vi "Load 1PLOT.vi"(8 "error in (no error)":errorcluster, 11 "Config Ops":T6={"file extension"="", "start path"=path ""}) -> (0 "error out":errorcluster, 2 "Valid load?":bool, 3 "Plot Config":T1={"plots"=[], "X-axis"={"Name Label.Text"="", "Style"=0, "Tick Colors:Minor Tick Color"=0, "Tick Colors:Tick Color"=0, "Marker Colors:Text Color"=0, "Grid Colors:Major Color"=0, "Grid Colors:Minor Color"=0, "Mapping Mode"=0, "Flipped"=FALSE, "Name Label.Visible"=FALSE, "Name Label.Text Colors:Text Color"=0, "Scale Fit"=0, "Range:Maximum"=0.0, "Range:Minimum"=0.0, "Offset and Multiplier:Multiplier"=0.0, "Offset and Multiplier:Offset"=0.0, "Name Label.Font:Size"=0, "Marker.Font:Size"=0, "Uniform Marker Spacing?"=TRUE, "Format String"=""}, "Y-axes"=[], "General"={"Title"="", "Time to Plot"=1800.0, "Title.Visible"=FALSE, "Sidebar.Visible"=FALSE, "Plot Area:Colors:BG Color"=0, "X Scale.Plot Name"="", "X Scale.Use Plot Name"=FALSE}} {"General"."Time to Plot" format="%<%M:%S>t"})   [LabVIEW 2021, in "RocketPlot.lvlib"]
uses:
  RocketPlot.lvlib
  TypeDefs/Save 1PLOT config.ctl
  TypeDefs/plot load data V2.ctl
  TypeDefs/plot properties V2.ctl
  TypeDefs/plot attributes V2.ctl
  TypeDefs/Plot scale axis properties.ctl
  TypeDefs/Plot general properties.ctl
  314c0d5c-2ca3-4b39-84aa-e4fa527c7e45.vi
  <vilib>/JDP Science/JSONtext/JSON text to Variant.vi
  <vilib>/JDP Science/JSONtext/LVClass Serializer/JSONtext LVClass Serializer.lvclass
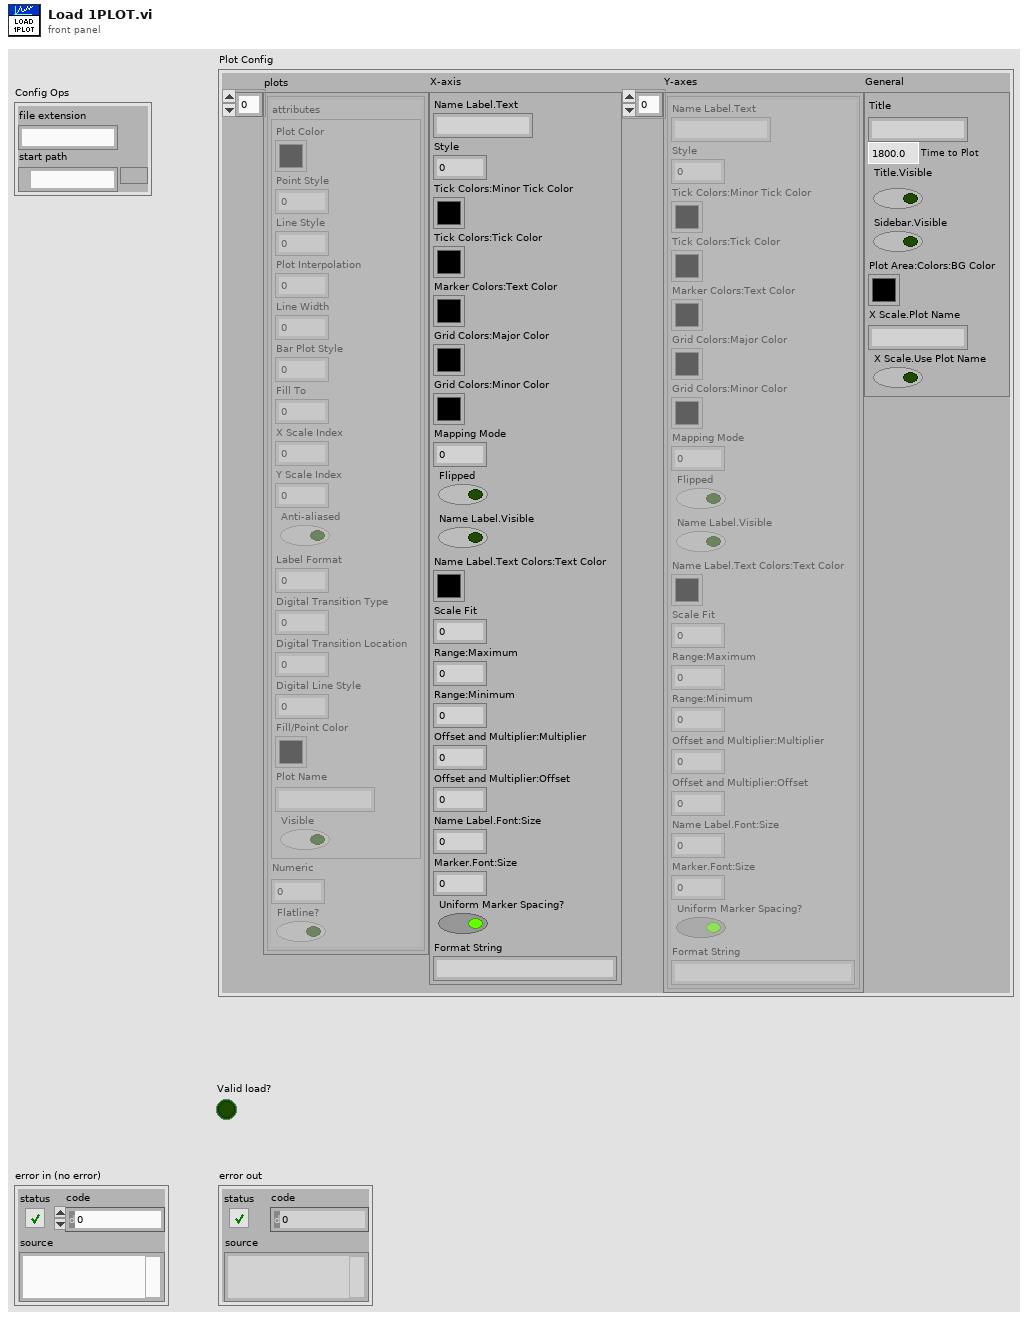
[diagram p1: front panel]
types:
  T1 = typedef "RocketPlot.lvlib/plot load data V2.ctl" = cluster{"plots":T2[], "X-axis":T4, "Y-axes":T4[], "General":T5}
  T2 = typedef "RocketPlot.lvlib/plot properties V2.ctl" = cluster{"attributes":T3, "Numeric":dbl, "Flatline?":bool}
  T3 = typedef "RocketPlot.lvlib/plot attributes V2.ctl" = cluster{"Plot Color":u32, "Point Style":u8, "Line Style":u8, "Plot Interpolation":u8, "Line Width":u8, "Bar Plot Style":u8, "Fill To":i16, "X Scale Index":u32, "Y Scale Index":u32, "Anti-aliased":bool, "Label Format":u8, "Digital Transition Type":u8, "Digital Transition Location":u8, "Digital Line Style":u8, "Fill/Point Color":u32, "Plot Name":string, "Visible":bool}
  T4 = typedef "RocketPlot.lvlib/Plot scale axis properties.ctl" = cluster{"Name Label.Text":string, "Style":u8, "Tick Colors:Minor Tick Color":u32, "Tick Colors:Tick Color":u32, "Marker Colors:Text Color":u32, "Grid Colors:Major Color":u32, "Grid Colors:Minor Color":u32, "Mapping Mode":u8, "Flipped":bool, "Name Label.Visible":bool, "Name Label.Text Colors:Text Color":u32, "Scale Fit":u8, "Range:Maximum":dbl, "Range:Minimum":dbl, "Offset and Multiplier:Multiplier":dbl, "Offset and Multiplier:Offset":dbl, "Name Label.Font:Size":u32, "Marker.Font:Size":u32, "Uniform Marker Spacing?":bool, "Format String":string}
  T5 = typedef "RocketPlot.lvlib/Plot general properties.ctl" = cluster{"Title":string, "Time to Plot":dbl, "Title.Visible":bool, "Sidebar.Visible":bool, "Plot Area:Colors:BG Color":u32, "X Scale.Plot Name":string, "X Scale.Use Plot Name":bool}
  T6 = typedef "RocketPlot.lvlib/Save 1PLOT config.ctl" = cluster{"file extension":string, "start path":path}
  T7 = enum16{"open", "replace", "create", "open or create", "replace or create", "replace or create with confirmation"}
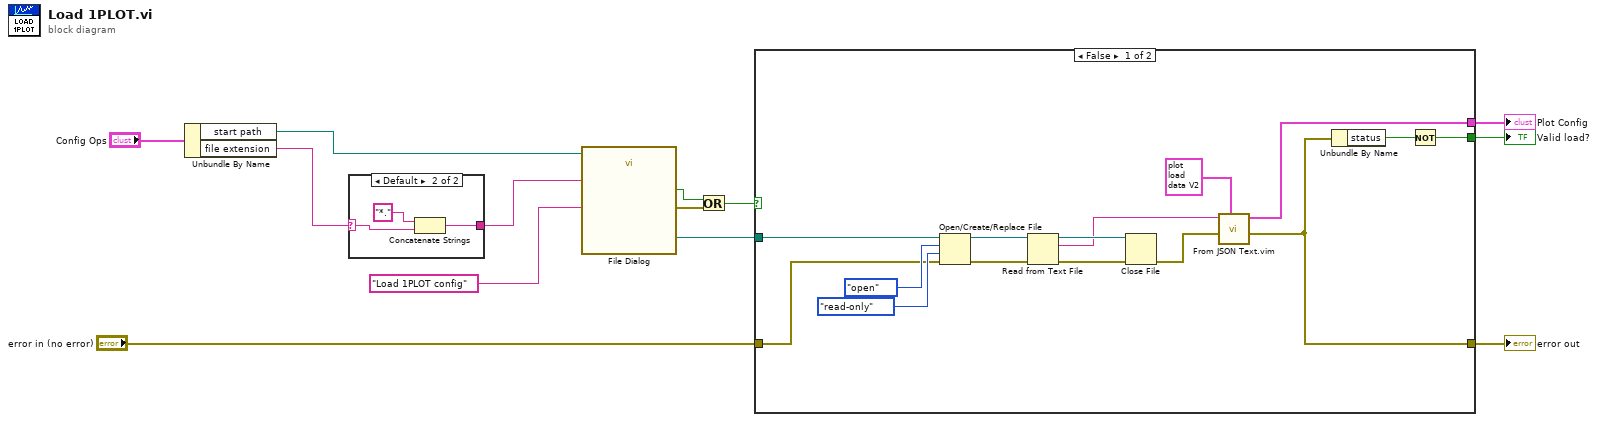
[diagram p0: block diagram]
diagram:
  n1 = Unbundle By Name("Config Ops") -> ("start path"=w12:path, "file extension"=w11:string)
  n2 = case shown="Default" w11 {
    selector: w11 -> [w14 w16]
    tunnel: [w14 w15] -> w10
    frame "" {
    }
    frame Default {
      n3 = Concatenate Strings("*." ("string"), w16) -> (w15:string)
    }
  }
  n4 = call "File Dialog"("start path"=w12, "prompt"="Load 1PLOT config", "pattern (all files)"=w10) -> ("selected path"=w5:path, "cancelled"=w8:bool, "error out"=w7:errorcluster)  [unwired: 9 in, 1 out]
  n5 = Or(x=w8, y=w7) -> (x .or. y?=w6:bool)
  n6 = case shown="False" w6 {
    tunnel: w5 -> [w24 _]
    tunnel: [w19 w33] -> w4
    tunnel: "error in (no error)" -> [w21 w33]
    tunnel: [w18 _] -> w2
    tunnel: [w31 _] -> w1
    frame False {
      n7 = Open/Create/Replace File(file path (use dialog)=w24, error in=w21, operation (0:open)=T7."open", access (0:read/write)=enum16{"read/write", "read-only", "write-only"}."read-only") -> (refnum out=w27:refnum<file>, error out=w29:errorcluster)  [unwired: 2 in, 1 out]
      n8 = Read from Text File(file (use dialog)=w27, error in=w29) -> (refnum out=w28:refnum<file>, text=w22:string, error out=w30:errorcluster)  [unwired: 2 in, 1 out]
      n9 = Close File(refnum=w28, error in=w30) -> (error out=w20:errorcluster)  [unwired: 1 out]
      n10 = call "From JSON Text.vim"("Data Type and Default Value"=T1 {"plots"=[], "X-axis"={"Name Label.Text"="", "Style"=0, "Tick Colors:Minor Tick Color"=0, "Tick Colors:Tick Color"=0, "Marker Colors:Text Color"=0, "Grid Colors:Major Color"=0, "Grid Colors:Minor Color"=0, "Mapping Mode"=0, "Flipped"=FALSE, "Name Label.Visible"=FALSE, "Name Label.Text Colors:Text Color"=0, "Scale Fit"=0, "Range:Maximum"=0.0, "Range:Minimum"=0.0, "Offset and Multiplier:Multiplier"=0.0, "Offset and Multiplier:Offset"=0.0, "Name Label.Font:Size"=0, "Marker.Font:Size"=0, "Uniform Marker Spacing?"=TRUE, "Format String"=""}, "Y-axes"=[], "General"={"Title"="", "Time to Plot"=1800.0, "Title.Visible"=FALSE, "Sidebar.Visible"=FALSE, "Plot Area:Colors:BG Color"=0, "X Scale.Plot Name"="", "X Scale.Use Plot Name"=FALSE}} ("SerializableData.Plot config"), "error in (no error)"=w20, "JSON"=w22) -> ("error out"=w19:errorcluster, "Data out"=w18:T1)  [unwired: 7 in]
      n11 = Unbundle By Name(w19) -> ("status"=w32:bool)
      n12 = Not(x=w32) -> (.not. x?=w31:bool)
    }
    frame True {
    }
  }
  "error out" <- w4
  "Plot Config" <- w2
  "Valid load?" <- w1
